vi "params.vi"   [LabVIEW 2012]
uses:
  <vilib>/addons/internet/NI_InternetTK_Core_VIs.lvlib
types:
  T1 = typedef "CGI Connection Info.ctl" = cluster{"name":string, "type":T2, "session":T3}
  T2 = typedef "CGI Request Type.ctl" = enum16{"cgi", ".spool first", ".spool", ".spool last"}
  T3 = typedef "HTTP Session.ctl" = refnum<k1>
  T4 = typedef "NI_FTP.lvlib/Keyed Array.ctl" = cluster{"keys":string[], "values":string[]}
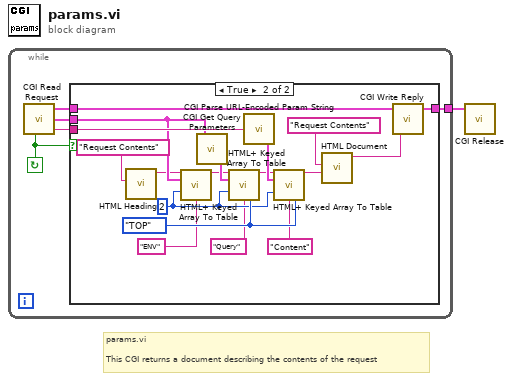
[diagram p0: block diagram]
diagram:
  # "params.vi\n\nThis CGI returns a document describing the contents of the request"
  n1 = while {
    tunnel: [w5] -> w1
    stop <- w4 continue-if-true
    n2 = call <vilib>:"CGI Read Request.vi"() -> ("valid request?"=w4:bool, "cgi connection info"=w6:T1, "env"=w3:T4, "content"=w2:string)  [unwired: 4 in]
    n3 = case shown="True" w4 {
      tunnel: [w7 w25] -> w5
      tunnel: w6 -> [w7 w24]
      tunnel: w3 -> [_ w15]
      tunnel: w2 -> [_ w21]
      frame False {
      }
      frame True {
        w22 = enum16{"(default)", "TOP", "BOTTOM"}."TOP" ("caption align (default)")
        w16 = 2 ("border width (default)")
        n4 = call <vilib>:"HTML Heading.vi"("heading"="Request Contents") -> ("HTML out"=w10:string)  [unwired: 10 in]
        n5 = call <vilib>:"HTML+ Keyed Array To Table.vi"("HTML in"=w10, "keyed array"=w15, "border width (default)"=w16, "caption"="ENV") -> ("HTML out"=w14:string)  [unwired: 11 in]
        n6 = call <vilib>:"CGI Get Query Parameters.vi"("env"=w15) -> ("query params"=w23:T4)  [unwired: 2 out]
        n7 = call <vilib>:"HTML+ Keyed Array To Table.vi"("HTML in"=w14, "keyed array"=w23, "border width (default)"=w16, "caption"="Query", "caption align (default)"=w22) -> ("HTML out"=w17:string)  [unwired: 10 in]
        n8 = call <vilib>:"CGI Parse URL-Encoded Param String.vi"("url-encoded param string"=w21) -> ("params"=w20:T4)
        n9 = call <vilib>:"HTML+ Keyed Array To Table.vi"("HTML in"=w17, "keyed array"=w20, "border width (default)"=w16, "caption"="Content", "caption align (default)"=w22) -> ("HTML out"=w19:string)  [unwired: 10 in]
        n10 = call <vilib>:"HTML Document.vi"("document body"=w19, "document title"="Request Contents") -> ("HTML Document"=w8:string)  [unwired: 9 in]
        n11 = call <vilib>:"CGI Write Reply.vi"("content"=w8, "cgi connection info"=w24) -> ("cgi connection info out"=w25:T1)  [unwired: 3 in]
      }
    }
  }
  n12 = call <vilib>:"CGI Release.vi"("cgi connection info"=w1) -> ()  [unwired: 5 in]
